vi "Write channel.vi"(8 "error in (no error)":errorcluster, 10 "channel":string, 11 "Abstract_Instrument in":refnum<class "Abstract_Instrument.lvclass">) -> (0 "error out":errorcluster, 3 "Abstract_Instrument out":refnum<class "Abstract_Instrument.lvclass">)   [LabVIEW 2021, in "Abstract_Instrument.lvclass"]
uses:
  Abstract_Instrument.lvclass
  Abstract_Instrument.lvclass/Abstract_Instrument.ctl
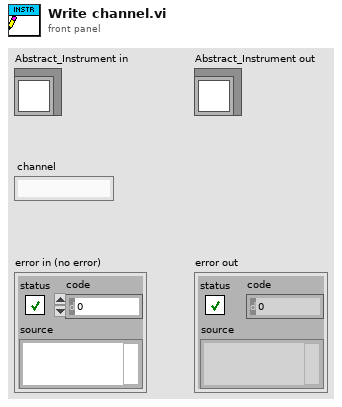
[diagram p1: front panel]
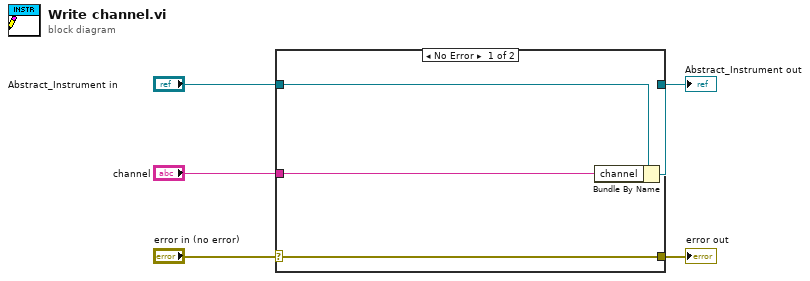
[diagram p0: block diagram]
diagram:
  n1 = case shown="No Error" "error in (no error)" {
    selector: "error in (no error)" -> [w9 w10]
    tunnel: [w9 w10] -> w4
    tunnel: [w7 w11] -> w2
    tunnel: "Abstract_Instrument in" -> [w8 w11]
    tunnel: "channel" -> [w6 _]
    frame No Error {
      n2 = Bundle By Name(cluster=w8, "channel"=w6) -> (w7:refnum<class "Abstract_Instrument.lvclass">)
    }
    frame Error {
    }
  }
  "error out" <- w4
  "Abstract_Instrument out" <- w2
